vi "MpembadDW.vi"(6 "Fmax":sgl, 7 "ktrap*mob":sgl, 8 "dE":sgl, 9 "Eb":sgl, 10 "Xm":sgl, 11 "Xpos":sgl) -> (2 "DWvolt":sgl, 3 "Force":sgl)   [LabVIEW 2019]
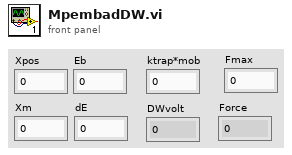
[diagram p1: front panel]
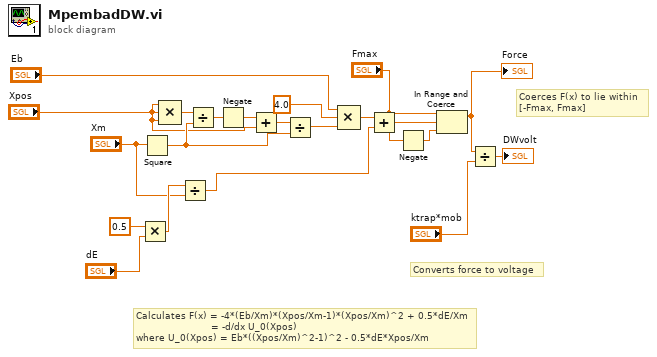
[diagram p0: block diagram]
diagram:
  # "Converts force to voltage"
  # "Coerces F(x) to lie within \n[-Fmax, Fmax]"
  # "Calculates F(x) = -4*(Eb/Xm)*(Xpos/Xm-1)*(Xpos/Xm)^2 + 0.5*dE/Xm\n                         = -d/dx U_0(Xpos) \nwhere U_0(Xpos) = Eb*((Xpos/Xm)^2-1)^2 - 0.5*dE*Xpos/Xm"
  n1 = Multiply(x=sgl 0.5 ("y"), y="dE") -> (x*y=w5:sgl)
  n2 = Square(x="Xm") -> (x^2=w16:sgl)
  n3 = Compound Arithmetic op=MULTIPLY("Xpos", "Xpos", "Xpos") -> (w18:sgl)
  n4 = Divide(x=w5, y="Xm") -> (x/y=w2:sgl)
  n5 = Divide(x=w18, y=w16) -> (x/y=w15:sgl)
  n6 = Negate(x=w15) -> (-x=w14:sgl)
  n7 = Add(x=w14, y="Xpos") -> (x+y=w17:sgl)
  n8 = Divide(x=w17, y=w16) -> (x/y=w21:sgl)
  n9 = Compound Arithmetic op=MULTIPLY("Eb", sgl 4.0 ("value"), w21) -> (w3:sgl)
  n10 = Add(x=w3, y=w2) -> (x+y=w1:sgl)
  n11 = Negate(x="Fmax") -> (-x=w11:sgl)
  n12 = In Range and Coerce(upper limit="Fmax", x=w1, lower limit=w11) -> (coerced(x)=w7:sgl)  [unwired: 1 out]
  "Force" <- w7
  n13 = Divide(x=w7, y="ktrap*mob") -> (x/y=→"DWvolt":sgl)
